vi "2P ready check.vi"(5 "Sample Clock Source":tag="OnboardClock", 6 "error in":errorcluster, 9 "Line(s)":tag="Dev1/port0/line0:7") -> (0 "error out":errorcluster)   [LabVIEW 2018]
uses:
  <vilib>/Utility/error.llb/DialogType.ctl
  <vilib>/DAQmx/read.llb/DAQmx Read (Digital 1D U32 1Chan NSamp).vi
  <vilib>/DAQmx/create/channels.llb/DAQmx Create Channel (DI-Digital Input).vi
  <vilib>/DAQmx/configure/timing.llb/DAQmx Timing (Sample Clock).vi
  <vilib>/DAQmx/miscellaneous.llb/DAQmx Fill In Error Info.vi
panel:
  in  "Number of Samples":i32=100
  in  "Sample Rate":dbl=1000.0
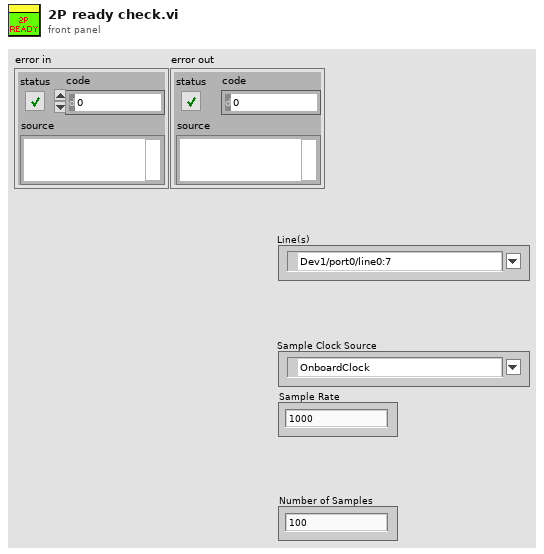
[diagram p1: front panel]
types:
  T1 = typedef "DialogType.ctl" = u16
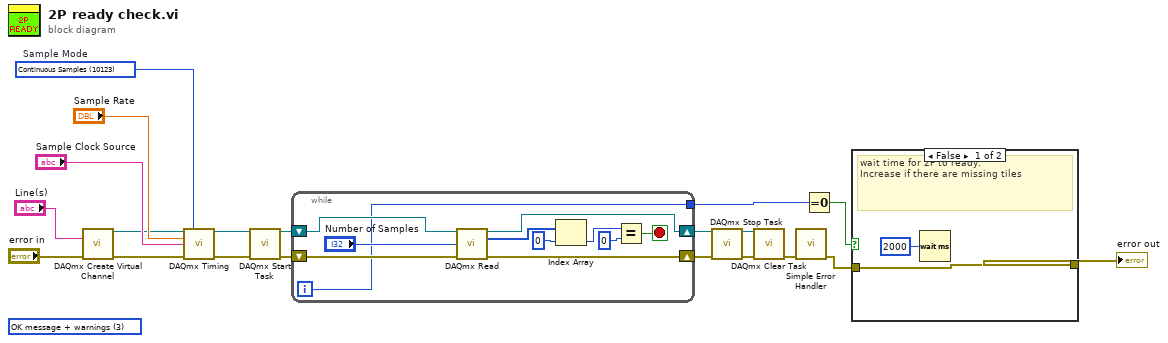
[diagram p0: block diagram]
diagram:
  (unwired) T1 3 items=["no dialog", "OK message", "continue or stop message", "OK message + warnings", "continue/stop + warnings"] ("type of dialog (OK msg:1)")
  w19 = 10123 items=["Finite Samples"=10178, "Continuous Samples"=10123, "Hardware Timed Single Point"=12522]  # Sample Mode
  n1 = call-poly <vilib>:"DAQmx Create Virtual Channel.vi"("lines"="Line(s)", "error in"="error in") -> ("task out"=w16:refnum<k21>, "error out"=w15:errorcluster)  [unwired: 12 in]
  n2 = call-poly <vilib>:"DAQmx Timing.vi"("task/channels in"=w16, "sample mode"=w19, "rate"="Sample Rate", "source"="Sample Clock Source", "error in"=w15) -> ("task out"=w13:refnum<k21>, "error out"=w14:errorcluster)  [unwired: 9 in]
  n3 = call <vilib>:"DAQmx Start Task.vi"("task/channels in"=w13, "error in"=w14) -> ("task out"=w8:refnum<k21>, "error out"=w9:errorcluster)  [unwired: 12 in]
  n4 = while {
    shift-right: [w27] -> w6
    shift-left: w9 -> [w30]
    shift-right: [w28] -> w7
    shift-left: w8 -> [w29]
    tunnel: [w21] -> w4
    i -> [w21]
    stop <- w22 stop-if-true
    n5 = call-poly <vilib>:"DAQmx Read.vi"("task/channels in"=w29, "number of samples per channel"="Number of Samples", "error in"=w30) -> ("task out"=w28:refnum<k21>, "data"=w26:u32[], "error out"=w27:errorcluster)  [unwired: 10 in]
    n6 = Index Array(array=w26, index=0) -> (element=w24:u32)
    n7 = Equal?(x=w24, y=u8 0) -> (x = y?=w22:bool)
  }
  n8 = call <vilib>:"DAQmx Stop Task.vi"("task/channels in"=w7, "error in"=w6) -> ("task out"=w11:refnum<k21>, "error out"=w5:errorcluster)  [unwired: 12 in]
  n9 = call <vilib>:"DAQmx Clear Task.vi"("task in"=w11, "error in"=w5) -> ("error out"=w10:errorcluster)  [unwired: 13 in]
  n10 = call <vilib>:"Simple Error Handler.vi"("error in (no error)"=w10) -> ("error out"=w2:errorcluster)  [unwired: 4 in, 4 out]
  n11 = Equal To 0?(x=w4) -> (x = 0?=w3:bool)
  n12 = case shown="False" w3 {
    tunnel: w2 -> [w32 w34]
    tunnel: [w32 w34] -> w1
    frame False {
      # "wait time for 2P to ready.\nIncrease if there are missing tiles"
      n13 = Wait (ms)(milliseconds to wait=u32 2000) -> ()  [unwired: 1 out]
    }
    frame True {
    }
  }
  "error out" <- w1
